vi "CheckWithinBounds.vi"(8 "Response Array":T1[](array[typedef]), 9 "Addresses to Search":string[](array[string]), 10 "Spawn Rate":i32) -> (2 "Pings to Spawn":i32)   [LabVIEW 2020, in "Controller.lvlib"]
uses:
  Controller.lvlib
  Public Controls/IP Address Response Type Def.ctl
  UI/UI.lvlib
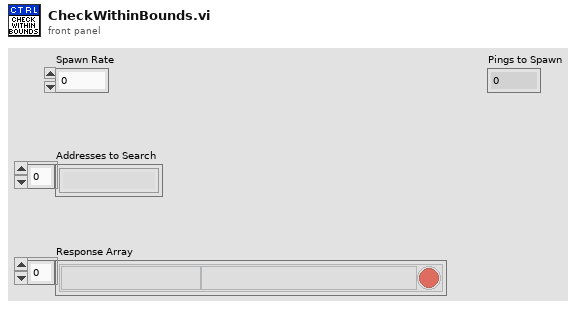
[diagram p1: front panel]
types:
  T1 = typedef "UI.lvlib/IP Address Response Type Def.ctl" = cluster{"Address":string, "Response":string, "Boolean":bool}
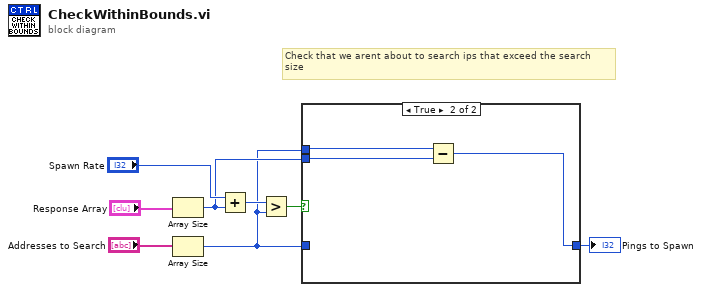
[diagram p0: block diagram]
diagram:
  # "Check that we arent about to search ips that exceed the search\nsize"
  n1 = Array Size(array="Response Array") -> (size(s)=w3:i32)
  n2 = Array Size(array="Addresses to Search") -> (size(s)=w2:i32)
  n3 = Add(x="Spawn Rate", y=w3) -> (x+y=w5:i32)
  n4 = Greater?(x=w5, y=w2) -> (0:w4:bool)
  n5 = case shown="True" w4 {
    tunnel: w2 -> [w9 _]
    tunnel: [w9 w10] -> w1
    tunnel: w3 -> [_ w11]
    tunnel: w2 -> [_ w12]
    frame False {
    }
    frame True {
      n6 = Subtract(x=w12, y=w11) -> (x-y=w10:i32)
    }
  }
  "Pings to Spawn" <- w1
